vi "read all temps.vi"(8 "error in (no error)":errorcluster, 11 "Thermocouples in":refnum<class "Thermocouples.lvclass">) -> (0 "error out":errorcluster, 2 "Temps":dbl[](array[numeric]) format="%0.2f", 3 "Thermocouples out":refnum<class "Thermocouples.lvclass">)   [LabVIEW 2025, in "Thermocouples.lvclass"]
uses:
  Thermocouples.lvclass
  Thermocouples.lvclass/Thermocouples.ctl
  <vilib>/DAQmx/read.llb/DAQmx Read (Analog 1D DBL NChan 1Samp).vi
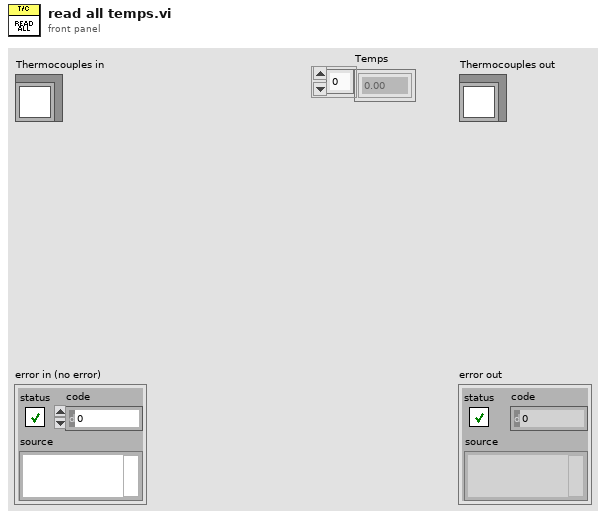
[diagram p1: front panel]
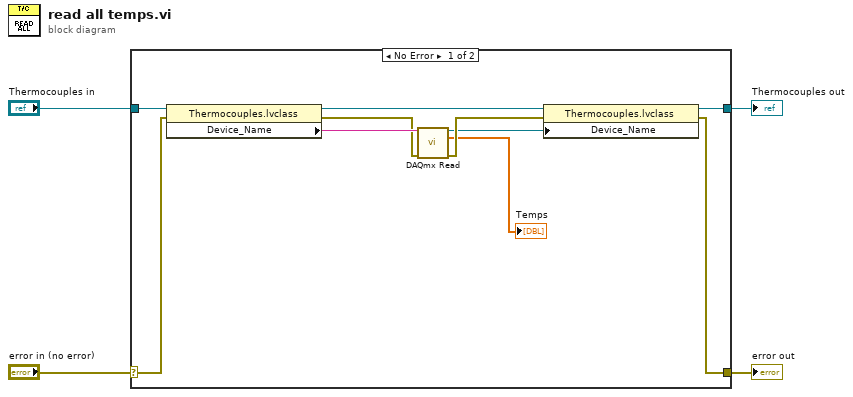
[diagram p0: block diagram]
diagram:
  n1 = case shown="No Error" "error in (no error)" {
    selector: "error in (no error)" -> [w13 w16]
    tunnel: [w6 w16] -> w3
    tunnel: [w7 w15] -> w1
    tunnel: "Thermocouples in" -> [w14 w15]
    frame No Error {
      n2 = property class="Thermocouples.lvclass"(reference=w14, error in=w13) -> (reference out=w10:refnum<class "Thermocouples.lvclass">, error out=w11:errorcluster, "Device_Name"=w12:string)
      n3 = call-poly <vilib>:"DAQmx Read.vi"("task/channels in"=w12, "error in"=w11) -> ("task out"=w8:refnum<k21>, "data"=→"Temps":dbl[], "error out"=w9:errorcluster)  [unwired: 11 in]
      n4 = property class="Thermocouples.lvclass"(reference=w10, error in=w9, "Device_Name"=w8) -> (reference out=w7:refnum<class "Thermocouples.lvclass">, error out=w6:errorcluster)
    }
    frame Error {
    }
  }
  "error out" <- w3
  "Thermocouples out" <- w1
